vi "EndEarly.vi"() -> ()   [LabVIEW 2021]
panel:
  out "endedEarly":bool
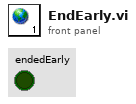
[diagram p1: front panel]
diagram:
